vi "Write Buffer Size.vi"(10 "DVR Pool Size":i32, 11 "Template in":refnum<class "Template.lvclass">) -> (3 "Template out":refnum<class "Template.lvclass">)   [LabVIEW 2020, in "Template.lvlib" / "Template.lvclass"]
doc: "Sets the DVR Buffer Size"
uses:
  Template.lvclass
  Template.lvclass/Template.ctl
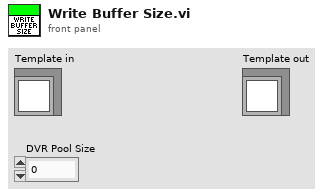
[diagram p1: front panel]
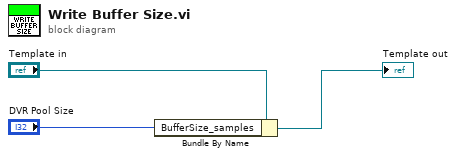
[diagram p0: block diagram]
diagram:
  n1 = Bundle By Name(cluster="Template in", "BufferSize_samples"="DVR Pool Size") -> (→"Template out":refnum<class "Template.lvclass">)
